vi "Clean CCD.vi"(8 "error in (no error)":errorcluster, 11 "CCDCamera in":refnum<class "CCDCamera.lvclass">) -> (0 "error out":errorcluster, 3 "CCDCamera out":refnum<class "CCDCamera.lvclass">)   [LabVIEW 2018, in "CCDCamera.lvclass"]
uses:
  CCDCamera.lvclass
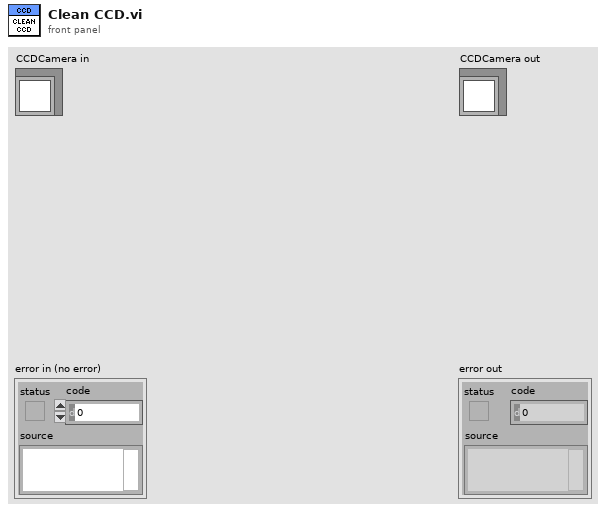
[diagram p1: front panel]
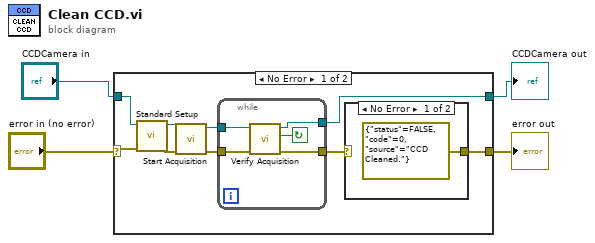
[diagram p0: block diagram]
diagram:
  n1 = case shown="No Error" "error in (no error)" {
    selector: "error in (no error)" -> [w5 w22]
    tunnel: "CCDCamera in" -> [w8 w21]
    tunnel: [w9 w21] -> w1
    tunnel: [w13 w22] -> w2
    frame No Error {
      n2 = call-dynamic "Standard Setup.vi"("error in (no error)"=w5, "CCDCamera in"=w8) -> ("error out"=w6:errorcluster, "CCDCamera out"=w7:refnum<class "CCDCamera.lvclass">)  [unwired: 8 in]
      n3 = call-dynamic "Start Acquisition.vi"("error in (no error)"=w6, "CCDCamera in"=w7) -> ("error out"=w11:errorcluster, "CCDCamera out"=w10:refnum<class "CCDCamera.lvclass">)  [unwired: 8 in]
      n4 = while {
        tunnel: [w19] -> w12
        tunnel: [w20] -> w9
        tunnel: w11 -> [w17]
        tunnel: w10 -> [w16]
        stop <- w18 continue-if-true
        n5 = call-dynamic "Verify Acquisition.vi"("error in (no error)"=w17, "CCDCamera in"=w16) -> ("error out"=w19:errorcluster, "Acquiring"=w18:bool, "CCDCamera out"=w20:refnum<class "CCDCamera.lvclass">)  [unwired: 7 in]
      }
      n6 = case shown="No Error" w12 {
        selector: w12 -> [_ w15]
        tunnel: [errorcluster {"status"=FALSE, "code"=0, "source"="CCD Cleaned."} ("error IO") w15] -> w13
        frame No Error {
        }
        frame Error {
        }
      }
    }
    frame Error {
    }
  }
  "error out" <- w2
  "CCDCamera out" <- w1
